vi "TDMS_read.vi"() -> ()   [LabVIEW 2011]
panel:
  out "data":dbl[](array[numeric])
  out "data 2":timestamp[](array[timestamp])
  out "error out":errorcluster
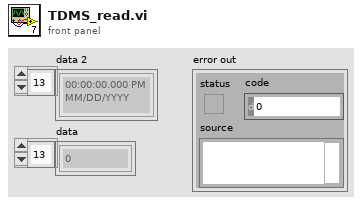
[diagram p1: front panel]
types:
  T1 = enum16{"open", "open or create", "create or replace", "create", "open (read-only)"}
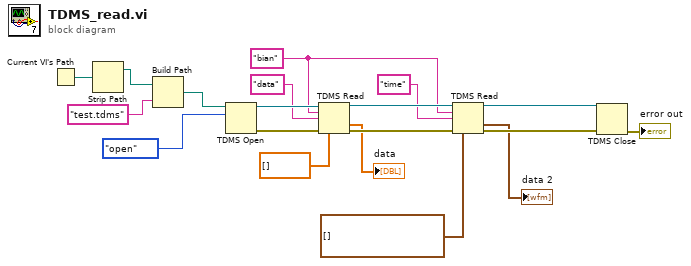
[diagram p0: block diagram]
diagram:
  w6 = "bian" ("group name in")
  n1 = Current VI's Path() -> (path=w19:path)
  n2 = Strip Path(path=w19) -> (stripped path=w18:path)  [unwired: 1 out]
  n3 = Build Path(base path=w18, name or relative path="test.tdms") -> (appended path=w16:path)
  n4 = TDMS Open(10:T1."open" ("operation (0:open)"), 11:w16) -> (0:w13:errorcluster, 3:w14:refnum<k34>)  [unwired: 4 in]
  n5 = TDMS Read(0:w14, 5:w6, 7:"data" ("group name in"), 11:w13, 12:dbl[] []) -> (4:w10:refnum<k34>, 10:→"data":dbl[], 15:w9:errorcluster)  [unwired: 3 in, 3 out]
  n6 = TDMS Read(0:w10, 5:w6, 7:"time" ("group name in"), 11:w9, 12:timestamp[] []) -> (4:w8:refnum<k34>, 10:→"data 2":timestamp[], 15:w7:errorcluster)  [unwired: 3 in, 3 out]
  n7 = TDMS Close(8:w7, 11:w8) -> (0:→"error out":errorcluster)  [unwired: 1 out]
